vi "Set Counter Settings--SubVI.vi"(8 "error in (no error)":errorcluster, 10 "Set Counter Settings Argument":T1, 11 "MB_Master_TCP in":refnum<class "MB_Master_TCP.lvclass">) -> (0 "error out":errorcluster, 3 "MB_Master_TCP out":refnum<class "MB_Master_TCP.lvclass">)   [LabVIEW 2024, in "FlexiFlowInterfaceCH2.lvlib"]
uses:
  FlexiFlowInterfaceCH2.lvlib
  <vilib>/Plasmionique/MB Master/MB_Master_TCP/MB_Master_TCP.lvclass
  Set Counter Settings Argument--cluster.ctl
  FlexiFlowDevice--enum.ctl
  Counter Settings--cluster.ctl
  Modbus Flexi-Flow API/Counter Setpoint Mode--enum.ctl
  Modbus Flexi-Flow API/Counter Modes--enum.ctl
  Modbus Flexi-Flow API/Bronkhorst Flexi-Flow ModbusTCP API.lvlib
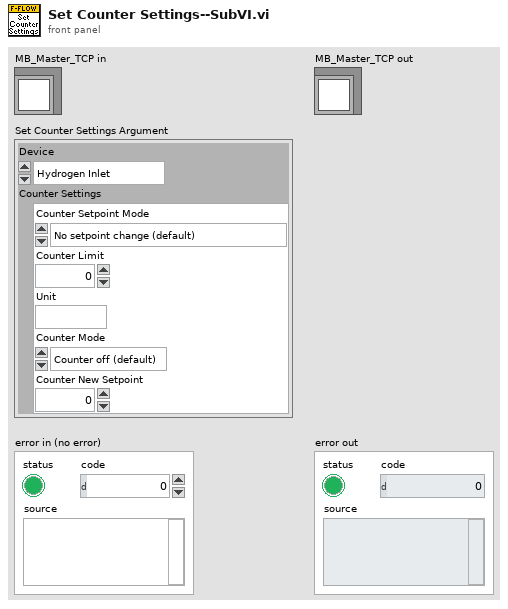
[diagram p1: front panel]
types:
  T1 = typedef "FlexiFlowInterfaceCH2.lvlib/Set Counter Settings Argument--cluster.ctl" = cluster{"Device":T2, "Counter Settings":T3}
  T2 = typedef "FlexiFlowInterfaceCH2.lvlib/FlexiFlowDevice--enum.ctl" = enum16{"Hydrogen Inlet", "Nitrogen Inlet", "Cathode Outlet", "Anode Outlet"}
  T3 = typedef "FlexiFlowInterfaceCH2.lvlib/Counter Settings--cluster.ctl" = cluster{"Counter Setpoint Mode":T4, "Counter Limit":sgl, "Unit":string, "Counter Mode":T5, "Counter New Setpoint":u16}
  T4 = typedef "Bronkhorst Flexi-Flow ModbusTCP API.lvlib/Counter Setpoint Mode--enum.ctl" = enum16{"No setpoint change (default)", "Change setpoint to Counter new setpoint"}
  T5 = typedef "Bronkhorst Flexi-Flow ModbusTCP API.lvlib/Counter Modes--enum.ctl" = enum16{"Counter off (default)", "Counting up continuously", "Counting up until limit reached"}
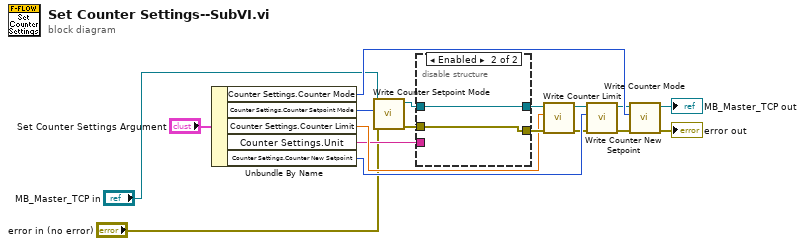
[diagram p0: block diagram]
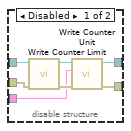
[diagram p2: hidden frame]
diagram:
  n1 = Unbundle By Name("Set Counter Settings Argument") -> ("Counter Settings.Counter Mode"=w9:T5, "Counter Settings.Counter Setpoint Mode"=w17:T4, "Counter Settings.Counter Limit"=w10:sgl, "Counter Settings.Unit"=w8:string, "Counter Settings.Counter New Setpoint"=w18:u16)
  n2 = call "Write Counter Setpoint Mode.vi"("error in"="error in (no error)", "Counter Setpoint Mode"=w17, "MB_TCP session in"="MB_Master_TCP in") -> ("error out"=w11:errorcluster, "MB session out"=w12:refnum<class "MB_Master_TCP.lvclass">)  [unwired: 6 in, 1 out]
  n3 = disable-structure shown="Enabled" {
    disable-tunnel: [w25 w27] -> w15
    disable-tunnel: [w24 w26] -> w13
    disable-tunnel: w12 -> [w21 w27]
    disable-tunnel: w11 -> [w20 w26]
    disable-tunnel: w8 -> [w19 _]
    frame Disabled {
      n4 = call "Write Counter Limit.vi"("error in"=w20, "MB_TCP session in"=w21) -> ("error out"=w23:errorcluster, "MB session out"=w22:refnum<class "MB_Master_TCP.lvclass">)  [unwired: 7 in, 1 out]
      n5 = call "Write Counter Unit.vi"("error in"=w23, "Unit"=w19, "MB_TCP session in"=w22) -> ("error out"=w24:errorcluster, "MB session out"=w25:refnum<class "MB_Master_TCP.lvclass">)  [unwired: 7 in]
    }
    frame Enabled {
    }
  }
  n6 = call "Write Counter Limit.vi"("error in"=w13, "Counter Limit"=w10, "MB_TCP session in"=w15) -> ("error out"=w14:errorcluster, "MB session out"=w16:refnum<class "MB_Master_TCP.lvclass">)  [unwired: 6 in, 1 out]
  n7 = call "Write Counter New Setpoint.vi"("error in"=w14, "New Setpoint Value"=w18, "MB_TCP session in"=w16) -> ("error out"=w5:errorcluster, "MB session out"=w6:refnum<class "MB_Master_TCP.lvclass">)  [unwired: 6 in, 1 out]
  n8 = call "Write Counter Mode.vi"("error in"=w5, "Counter Mode"=w9, "MB_TCP session in"=w6) -> ("error out"=→"error out":errorcluster, "MB session out"=→"MB_Master_TCP out":refnum<class "MB_Master_TCP.lvclass">)  [unwired: 7 in]
